vi "DealerDraw.vi"(2 "Number of decks":i32, 4 "Input dealer's cards":i32[](array[numeric]), 5 "Input used cards":i32[](array[numeric])) -> (0 "Output dealer's cards":i32[](array[numeric]), 1 "Output used cards":i32[](array[numeric]))   [LabVIEW 2018]
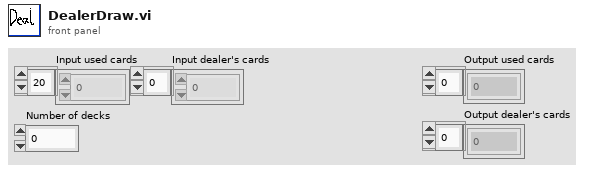
[diagram p1: front panel]
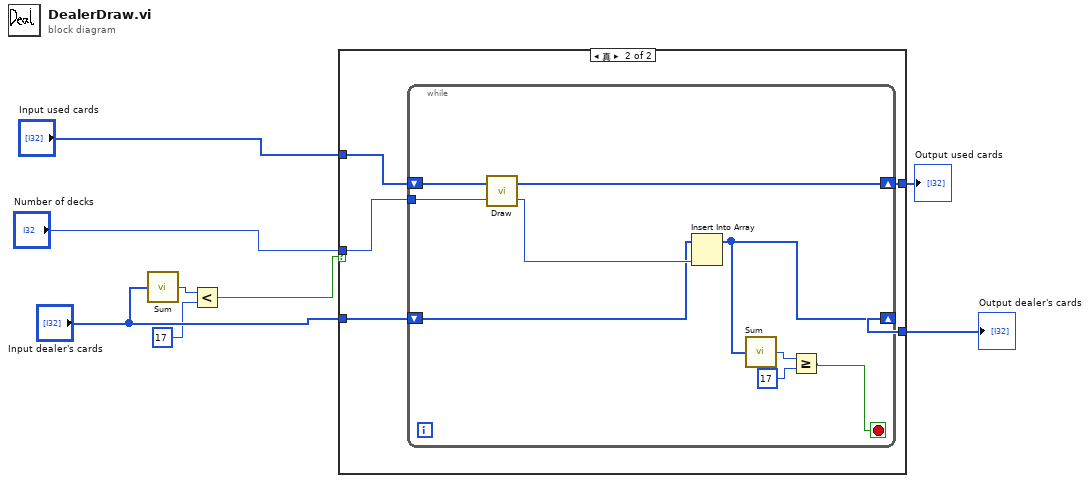
[diagram p0: block diagram]
diagram:
  n1 = call "Sum.vi"("Array"="Input dealer's cards") -> ("Value"=w3:i32)
  n2 = Less?(x=w3, y=17) -> (x < y?=w1:bool)
  n3 = case shown="真" w1 {
    tunnel: "Input used cards" -> [w9 w15]
    tunnel: [w9 w14] -> w7
    tunnel: "Number of decks" -> [_ w13]
    tunnel: "Input dealer's cards" -> [w10 w12]
    tunnel: [w10 w11] -> w5
    frame False {
    }
    frame True {
      n4 = while {
        shift-right: [w23] -> w14
        shift-left: w15 -> [w24]
        tunnel: w13 -> [w22]
        shift-right: [w19] -> w11
        shift-left: w12 -> [w20]
        stop <- w16 stop-if-true
        n5 = call "Draw.vi"("Number of decks"=w22, "Input used cards"=w24) -> ("No. of card"=w21:i32, "Output used cards"=w23:i32[])
        n6 = Insert Into Array(array=w20, new element=w21) -> (w19:i32[])  [unwired: 1 in]
        n7 = call "Sum.vi"("Array"=w19) -> ("Value"=w18:i32)
        n8 = Greater Or Equal?(x=w18, y=17) -> (x >= y?=w16:bool)
      }
    }
  }
  "Output used cards" <- w7
  "Output dealer's cards" <- w5
